vi "new Norm.vi"(8 "Fehler (Eingang, kein Fehler)":errorcluster, 11 "Data":T2={"Report.lvclass"=refnum, "Norm"="", "last State"=enum."Initialize", "Norm ID"=0, "parameter"=[], "EMTestCWS500N.lvclass"=refnum, "CEG4500.lvclass"=refnum, "Tektronix RSA5106A.lvclass"=refnum, "erfolgreich"=FALSE, "log"="", "Kommentar"="", "Device Enum"=enum."emTestCWS500N", "Test Enum"=enum."HF-Felder", "debug"=FALSE, "tab"=enum."Hauptmenü", "ESD Pistol.lvclass"=refnum}) -> (0 "Fehler (Ausgang)":errorcluster, 3 "Next State":T1=enum."enter Report Parameters")   [LabVIEW 2013, in "DataCreation.lvlib"]
uses:
  lib/DataCreation.lvlib
  Main/controls/Data.ctl
  classes/Datastructure/Report/Report.lvclass
  classes/Devices/emTestCWS500N/EMTestCWS500N.lvclass
  classes/Devices/CEG4500/CEG4500.lvclass
  classes/Devices/Tektronix RSA5106A/Tektronix RSA5106A.lvclass
  ESD Pistol.lvclass
  Main/controls/State.ctl
  classes/Devices/DeviceInterface/Devices.ctl
  classes/Tests/TestInterface/Tests.ctl
  Tabs.ctl
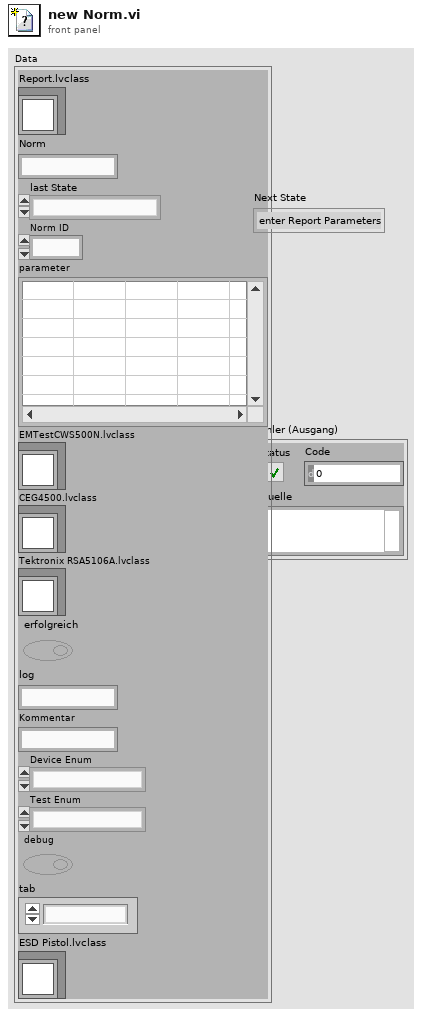
[diagram p1: front panel]
types:
  T1 = typedef "State.ctl" = enum16{"create Pdf", "load Report", "save Report", "do Test", "CDN Kalibrierung", "enter Report Parameters", "new Test", "Protokoll", "read Tree", "update Tree", "Fehler", "Initialize", "Wait for Event", "Exit"}
  T2 = typedef "Data.ctl" = cluster{"Report.lvclass":refnum<class "Report.lvclass">, "Norm":string, "last State":T1, "Norm ID":i32, "parameter":string[][], "EMTestCWS500N.lvclass":refnum<class "EMTestCWS500N.lvclass">, "CEG4500.lvclass":refnum<class "CEG4500.lvclass">, "Tektronix RSA5106A.lvclass":refnum<class "Tektronix RSA5106A.lvclass">, "erfolgreich":bool, "log":string, "Kommentar":string, "Device Enum":T3, "Test Enum":T4, "debug":bool, "tab":T5, "ESD Pistol.lvclass":refnum<class "ESD Pistol.lvclass">}
  T3 = typedef "Devices.ctl" = enum16{"unbekannt", "ESD Pistol", "Tektronix RSA5106A", "emTestCWS500N", "CEG-4500"}
  T4 = typedef "Tests.ctl" = enum16{"unbekannt", "Störaussendung", "Burst", "ESD", "Surge", "Spannungseinbruch", "HF-Felder"}
  T5 = typedef "Tabs.ctl" = enum32{"Hauptmenü", "Prüfbericht", "Einstellungen"}
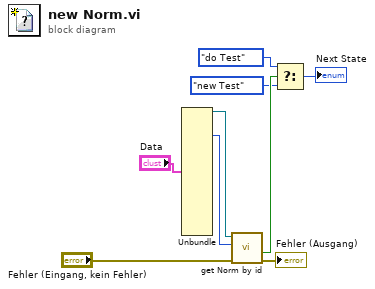
[diagram p0: block diagram]
diagram:
  n1 = Unbundle("Data") -> ("Report.lvclass"=w6:refnum<class "Report.lvclass">, "Norm ID"=w8:i32)  [unwired: 14 out]
  n2 = call-dynamic "get Norm by id.vi"("error in (no error)"="Fehler (Eingang, kein Fehler)", "id"=w8, "Report (Eingang)"=w6) -> ("error out"=→"Fehler (Ausgang)":errorcluster, "id found"=w4:bool)  [unwired: 4 in, 3 out]
  n3 = Select(t=State."do Test" ("Next State"), s=w4, f=State."new Test" ("Next State")) -> (s? t:f=→"Next State":T1)
